vi "CH_LM Config USB Streaming.vi"(0 "Meter Index":i32, 2 "USB Streaming (disable)":bool, 5 "error in (no error)":errorcluster, 7 "Timeout / ms (3000)":i32=3000, 8 "Action (query)":bool, 9 "Lock Timeout / ms (1000)":i32=1000) -> (11 "Lock timed out":bool, 14 "Meter Index":i32, 16 "USB Streaming":bool, 19 "error out":errorcluster)   [LabVIEW 2017, in "CH_LM.lvlib"]
doc: "This VI set/queries the status of USB Binary Data Streaming.\n\n<B>Hint:</B> Set command will be changed to query in case of non-USB communication mode."
uses:
  CH_LM.lvlib
  CH_LM Communication Mode.ctl
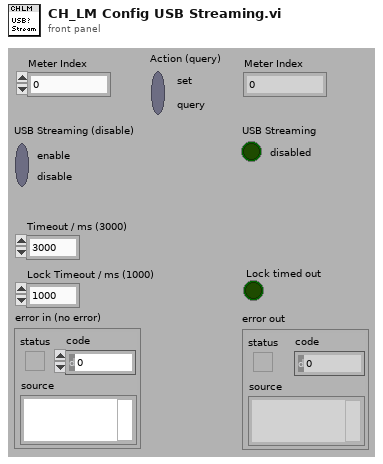
[diagram p1: front panel]
types:
  T1 = typedef "CH_LM.lvlib/CH_LM Communication Mode.ctl" = enum16{"None", "USB", "GPIB", "RS232"}
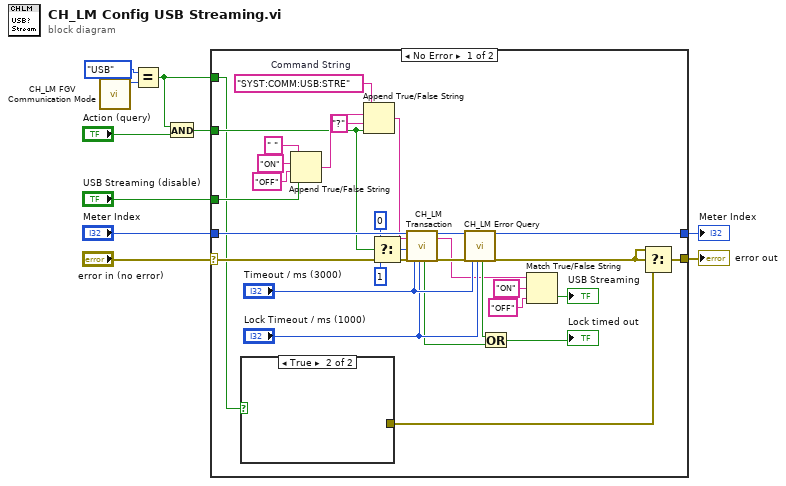
[diagram p0: block diagram]
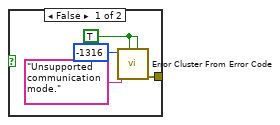
[diagram p2: hidden frame]
diagram:
  n1 = call "CH_LM FGV Communication Mode.vi"() -> ("Communication Mode"=w4:T1)  [unwired: 3 in, 5 out]
  n2 = Equal?(x=CH_LM_Communication_Mode."USB" ("Communication Mode"), y=w4) -> (x = y?=w1:bool)
  n3 = And(x=w1, y="Action (query)") -> (x .and. y?=w2:bool)
  n4 = case shown="No Error" "error in (no error)" {
    selector: "error in (no error)" -> [w40 w46]
    tunnel: [w12 w46] -> w10
    tunnel: "Meter Index" -> [w39 w45]
    tunnel: [w38 w45] -> w8
    tunnel: "USB Streaming (disable)" -> [w30 _]
    tunnel: w2 -> [w22 _]
    tunnel: w1 -> [w14 _]
    frame No Error {
      w27 = "SYST:COMM:USB:STRE"  # Command String
      n5 = case shown="True" w14 {
        tunnel: [w41 _] -> w11
        frame False {
          w42 = TRUE ("show call chain? (False)")
          n6 = call <vilib>:"Error Cluster From Error Code.vi"("is warning? (False)"=w42, "show call chain? (False)"=w42, "error message (\"\")"="Unsupported communication mode." ("error message (\"\")"), "error code (0)"=-1316) -> ("error out"=w41:errorcluster)  [unwired: 1 in, 4 out]
        }
        frame True {
        }
      }
      n7 = Append True/False String(1:w30, 2:"OFF" ("false string"), 3:"ON" ("true string"), 4:" " ("string (\"\")")) -> (0:w24:string)
      n8 = Append True/False String(1:w22, 2:"?", 3:w24, 4:w27) -> (0:w23:string)
      n9 = Select(t=0, s=w22, f=1) -> (s? t:f=w20:i32)
      n10 = call "CH_LM Transaction.vi"("Meter Index"=w39, "Command String"=w23, "NofStrings (-1:all)"=w20, "error in (no error)"=w40, "Timeout / ms (3000)"="Timeout / ms (3000)", "Lock Timeout / ms (1000)"="Lock Timeout / ms (1000)") -> ("Lock timed out"=w32:bool, "Meter Index"=w35:i32, "Response"=w17:string, "error out"=w34:errorcluster)  [unwired: 10 out]
      n11 = call "CH_LM Error Query.vi"("Meter Index"=w35, "error in (no error)"=w34, "Timeout / ms (3000)"="Timeout / ms (3000)", "Lock Timeout / ms (1000)"="Lock Timeout / ms (1000)") -> ("Lock timed out"=w33:bool, "Meter Index"=w38:i32, "error out"=w13:errorcluster)  [unwired: 13 out]
      n12 = Or(x=w33, y=w32) -> (x .or. y?=→"Lock timed out":bool)
      n13 = Match True/False String(2:"OFF" ("false string"), 3:"ON" ("true string"), 4:w17) -> (0:→"USB Streaming":bool)  [unwired: 1 out]
      n14 = Select(t=w13, s=w13, f=w11) -> (s? t:f=w12:errorcluster)
    }
    frame Error {
    }
  }
  "error out" <- w10
  "Meter Index" <- w8
